vi "getIDs.vi"(8 "error in (no error)":errorcluster, 11 "LLNode in":refnum<class "LLNode.lvclass">) -> (0 "error out":errorcluster, 2 "IDs":u32[](array[numeric]), 3 "LLNode out":refnum<class "LLNode.lvclass">)   [LabVIEW 2009, in "LLNode.lvclass"]
uses:
  LLNode.lvclass
  Node/Node.lvclass
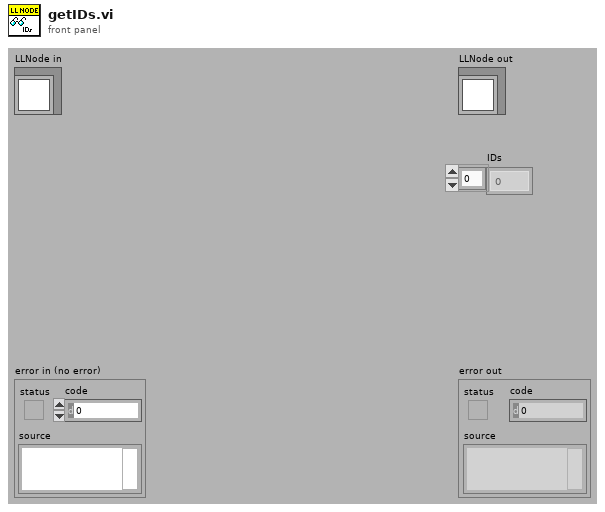
[diagram p1: front panel]
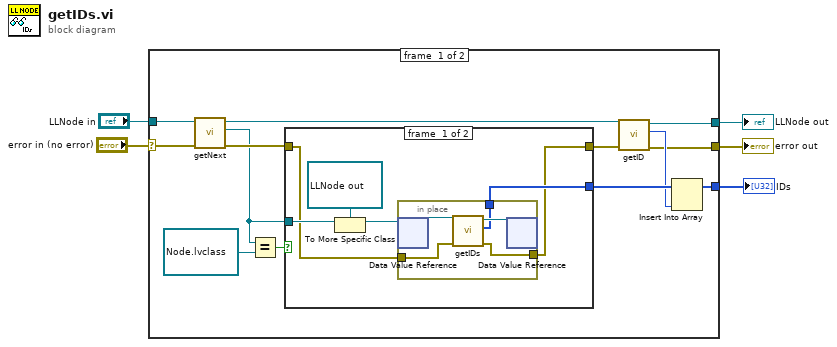
[diagram p0: block diagram]
diagram:
  n1 = case shown="No Error" "error in (no error)" {
    selector: "error in (no error)" -> [w17 w32]
    tunnel: [w7 w32] -> w4
    tunnel: [w9 w31] -> w2
    tunnel: "LLNode in" -> [w18 w31]
    tunnel: [w6 _] -> w1
    frame #0 {
      n2 = call "getNext.vi"("error in (no error)"=w17, "LLNode in"=w18) -> ("error out"=w14:errorcluster, "next"=w13:refnum<data-value>, "LLNode out"=w8:refnum<class "LLNode.lvclass">)  [unwired: 7 in]
      n3 = Equal?(x=w13, y=refnum<data-value> refnum) -> (x = y?=w15:bool)
      n4 = case shown="False" w15 {
        tunnel: w14 -> [w21 w30]
        tunnel: [w20 _] -> w11
        tunnel: [w19 w30] -> w12
        tunnel: w13 -> [w24 _]
        frame #0 {
          n5 = To More Specific Class(target class=refnum<data-value> refnum ("data value reference"), reference=w24) -> (specific class reference=w22:refnum<data-value>)  [unwired: 1 in, 1 out]
          n6 = in-place {
            in-place-border: w21 -> [w27]
            in-place-border: [w26] -> w19
            in-place-border: [w25] -> w20
            n7 = in-place-dvr #1(w22) -> (w29:refnum<class "LLNode.lvclass">)  [unwired: 1 out]
            n8 = call "getIDs.vi"("error in (no error)"=w27, "LLNode in"=w29) -> ("error out"=w26:errorcluster, "IDs"=w25:u32[], "LLNode out"=w28:refnum<class "LLNode.lvclass">)  [unwired: 7 in]
            n9 = in-place-dvr #1(w28) -> ()  [unwired: 2 out]
          }
        }
        frame #1 {
        }
      }
      n10 = call "getID.vi"("error in (no error)"=w12, "Node in"=w8) -> ("error out"=w7:errorcluster, "ID"=w10:u32, "Node out"=w9:refnum<class "LLNode.lvclass">)  [unwired: 7 in]
      n11 = Insert Into Array(array=w11, new element=w10) -> (w6:u32[])  [unwired: 1 in]
    }
    frame #1 {
    }
  }
  "error out" <- w4
  "LLNode out" <- w2
  "IDs" <- w1
